vi "Set PowerState.vi"(8 "error in (no error)":errorcluster, 10 "PowerState":enum16{"Off", "Sleep", "On"}(ring)=enum."Sleep", 11 "CellPhone in":refnum<class "CellPhone.lvclass">) -> (0 "error out":errorcluster, 3 "CellPhone out":refnum<class "CellPhone.lvclass">)   [LabVIEW 2009, in "CellPhone.lvclass"]
uses:
  CellPhone.lvclass
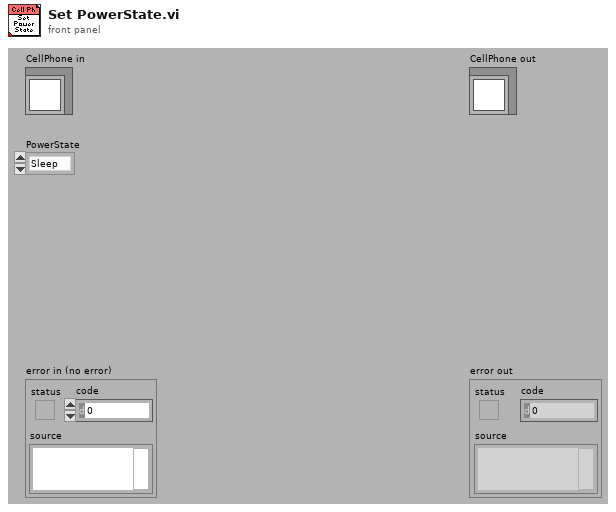
[diagram p1: front panel]
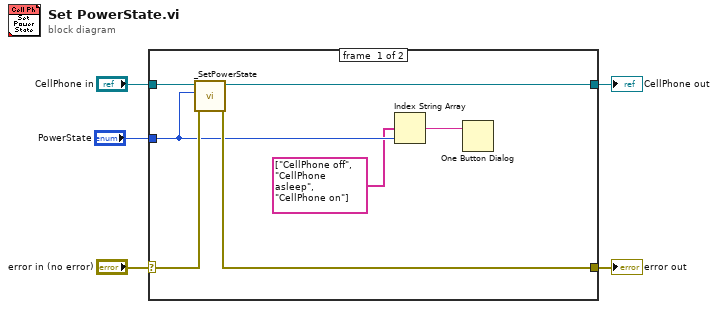
[diagram p0: block diagram]
diagram:
  n1 = case shown="No Error" "error in (no error)" {
    selector: "error in (no error)" -> [w10 w13]
    tunnel: [w9 w13] -> w4
    tunnel: [w11 w14] -> w2
    tunnel: "CellPhone in" -> [w12 w14]
    tunnel: "PowerState" -> [w8 _]
    frame #0 {
      n2 = call "_SetPowerState.vi"("error in (no error)"=w10, "PowerState"=w8, "CellPhone in"=w12) -> ("error out"=w9:errorcluster, "CellPhone out"=w11:refnum<class "CellPhone.lvclass">)  [unwired: 7 in]
      n3 = Index String Array(1:w8, 2:string[] ["CellPhone off", "CellPhone asleep", "CellPhone on"]) -> (0:w6:string)  [unwired: 1 in]
      n4 = One Button Dialog(message=w6) -> ()  [unwired: 1 in, 1 out]
    }
    frame #1 {
    }
  }
  "error out" <- w4
  "CellPhone out" <- w2
